vi "Homework#2.vi"() -> ()   [LabVIEW 2011]
panel:
  in  "Ranbow World":bool
  in  "stop":bool
  out "Time Step":dbl(slide) min=0.0 max=1000.0 scale=0.0..0.03 scale format="%#_2e"
  in  "Step Divisions":i32(slide)=1000 caption="Slide" min=600 max=1000000 scale=600.0..1000000.0
  in  "Starting Velocity":dbl(knob) scale=0.0..50.0
  in  "Starting Position":dbl(knob)=-3.0 scale=-100.0..100.0
  in  "Max Time(sec)":dbl(knob)=30.0 scale=0.0..300.0
  out "Van Derpol Forced Equation":cluster{"Y":dbl[], "Y":dbl[]}[](graph)
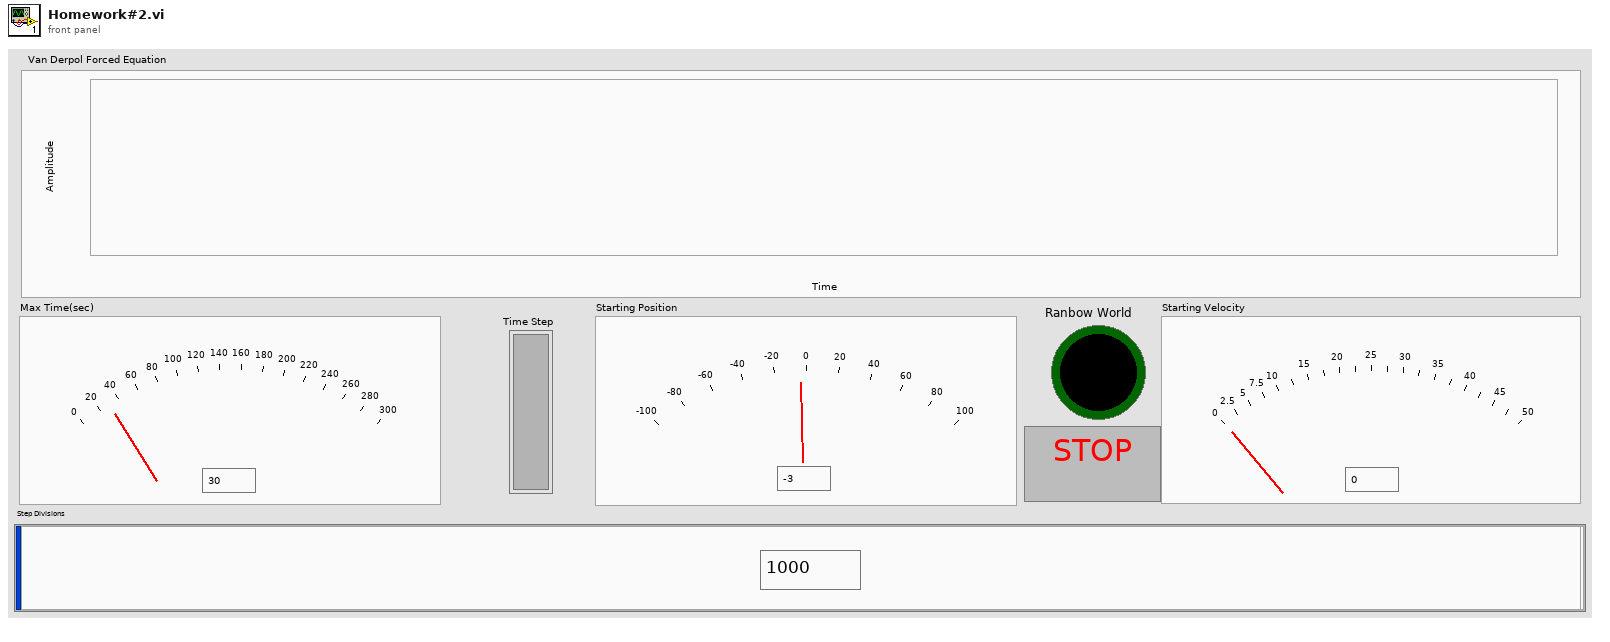
[diagram p1: front panel]
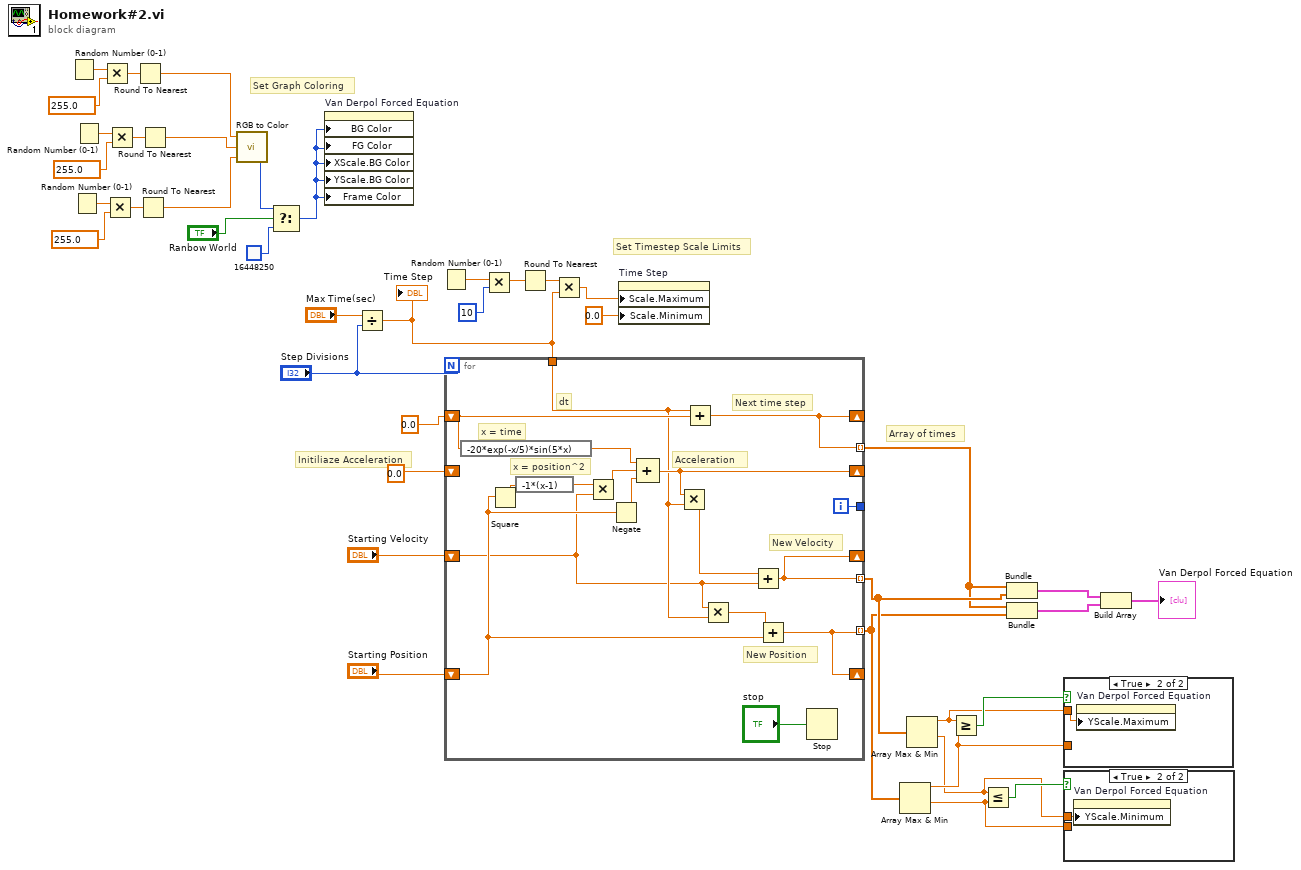
[diagram p0: block diagram]
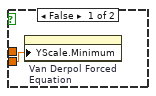
[diagram p2: hidden frame]
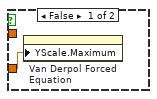
[diagram p3: hidden frame]
diagram:
  # "Array of times"
  # "Initiliaze Acceleration"
  # "Set Timestep Scale Limits"
  # "Set Graph Coloring"
  n1 = Random Number (0-1)() -> (number: 0 to 1=w35:dbl)
  n2 = Random Number (0-1)() -> (number: 0 to 1=w30:dbl)
  n3 = Random Number (0-1)() -> (number: 0 to 1=w31:dbl)
  n4 = Multiply(x=w35, y=255.0) -> (x*y=w33:dbl)
  n5 = Multiply(x=w30, y=255.0) -> (x*y=w29:dbl)
  n6 = Multiply(x=w31, y=255.0) -> (x*y=w32:dbl)
  n7 = Round To Nearest(number=w33) -> (nearest integer value=w24:dbl)
  n8 = Round To Nearest(number=w29) -> (nearest integer value=w25:dbl)
  n9 = Round To Nearest(number=w32) -> (nearest integer value=w26:dbl)
  n10 = call <vilib>:"RGB to Color.vi"("B"=w25, "G"=w26, "R"=w24) -> ("Color"=w2:u32)
  n11 = Select(t=w2, s="Ranbow World", f=u32 16448250) -> (s? t:f=w1:u32)
  n12 = property on="Van Derpol Forced Equation" class="XYGraph (strict)"("BG Color"=w1, "FG Color"=w1, "XScale.BG Color"=w1, "YScale.BG Color"=w1, "Frame Color"=w1) -> ()  [unwired: 2 in, 2 out]
  n13 = Divide(x="Max Time(sec)", y="Step Divisions") -> (x/y=w20:dbl)
  "Time Step" <- w20
  n14 = Random Number (0-1)() -> (number: 0 to 1=w39:dbl)
  n15 = for {
    N: "Step Divisions" -> [_]
    tunnel: [w58] -> w8 mode=indexing
    shift-right: [w58] -> _
    shift-left: 0.0 -> [w54]
    tunnel: [w55] -> w9 mode=indexing
    tunnel: [w56] -> w10 mode=indexing
    shift-right: [w55] -> _
    shift-left: "Starting Position" -> [w44]
    shift-right: [w56] -> _
    shift-left: "Starting Velocity" -> [w42]
    tunnel: w20 -> [w47]
    shift-right: [w49] -> _
    shift-left: 0.0 -> [_]
    tunnel: [w43] -> _
    i -> [w43]
    # "Acceleration"
    # "x = position^2"
    # "x = time"
    # "Next time step"
    # "dt"
    # "New Position"
    # "New Velocity"
    n16 = expression code="-20*exp(-x/5)*sin(5*x)"(w54) -> (w50:dbl)
    n17 = Square(x=w44) -> (x^2=w45:dbl)
    n18 = expression code="-1*(x-1)"(w45) -> (w53:dbl)
    n19 = Multiply(x=w53, y=w42) -> (x*y=w51:dbl)
    n20 = Negate(x=w44) -> (-x=w52:dbl)
    n21 = Compound Arithmetic op=ADD(w50, w51, w52) -> (w49:dbl)
    n22 = Multiply(x=w49, y=w47) -> (x*y=w48:dbl)
    n23 = Add(x=w47, y=w54) -> (x+y=w58:dbl)
    n24 = Multiply(x=w42, y=w47) -> (x*y=w46:dbl)
    n25 = Add(x=w48, y=w42) -> (x+y=w56:dbl)
    n26 = Add(x=w46, y=w44) -> (x+y=w55:dbl)
    n27 = Stop(stop? (T)="stop") -> ()
  }
  n28 = Multiply(x=w39, y=10) -> (x*y=w37:dbl)
  n29 = Round To Nearest(number=w37) -> (nearest integer value=w36:dbl)
  n30 = Multiply(x=w36, y=w20) -> (x*y=w40:dbl)
  n31 = property on="Time Step" class="Slide (strict)"("Scale.Maximum"=w40, "Scale.Minimum"=0.0) -> ()  [unwired: 2 in, 2 out]
  n32 = Array Max & Min(array=w9) -> (max value=w15:dbl, min value=w12:dbl)  [unwired: 2 out]
  n33 = Array Max & Min(array=w10) -> (max value=w16:dbl, min value=w13:dbl)  [unwired: 2 out]
  n34 = Greater Or Equal?(x=w16, y=w15) -> (x >= y?=w17:bool)
  n35 = Less Or Equal?(x=w13, y=w12) -> (x <= y?=w14:bool)
  n36 = Bundle(w8, w10) -> (w7:cluster{dbl[], dbl[]})  [unwired: 1 in]
  n37 = Bundle(w8, w9) -> (w6:cluster{dbl[], dbl[]})  [unwired: 1 in]
  n38 = case shown="True" w17 {
    tunnel: w16 -> [_ w60]
    tunnel: w15 -> [w59 _]
    frame False {
      n39 = property on="Van Derpol Forced Equation" class="XYGraph (strict)"("YScale.Maximum"=w59) -> ()  [unwired: 2 in, 2 out]
    }
    frame True {
      n40 = property on="Van Derpol Forced Equation" class="XYGraph (strict)"("YScale.Maximum"=w60) -> ()  [unwired: 2 in, 2 out]
    }
  }
  n41 = case shown="True" w14 {
    tunnel: w13 -> [_ w62]
    tunnel: w12 -> [w61 _]
    frame False {
      n42 = property on="Van Derpol Forced Equation" class="XYGraph (strict)"("YScale.Minimum"=w61) -> ()  [unwired: 2 in, 2 out]
    }
    frame True {
      n43 = property on="Van Derpol Forced Equation" class="XYGraph (strict)"("YScale.Minimum"=w62) -> ()  [unwired: 2 in, 2 out]
    }
  }
  n44 = Build Array(w7, w6) -> (→"Van Derpol Forced Equation":cluster{dbl[], dbl[]}[])
